vi "Initialize UI.vi"(8 "error in (no error)":errorcluster, 11 "UI in":refnum<class "UI.lvclass">) -> (0 "error out":errorcluster, 2 "stop event":refnum<user-event>, 3 "UI out":refnum<class "UI.lvclass">)   [LabVIEW 2016, in "Generic UI Actor.lvlib" / "UI.lvclass"]
uses:
  UI.lvclass
  UI.lvclass/UI.ctl
  Accessors/Write This VI.vi
  Accessors/Read This VI.vi
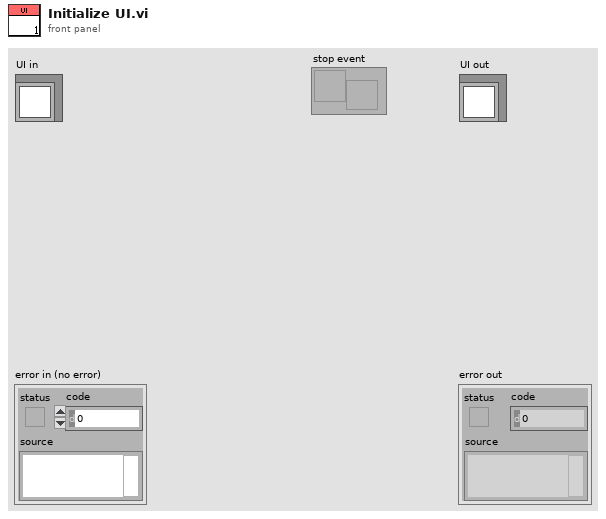
[diagram p1: front panel]
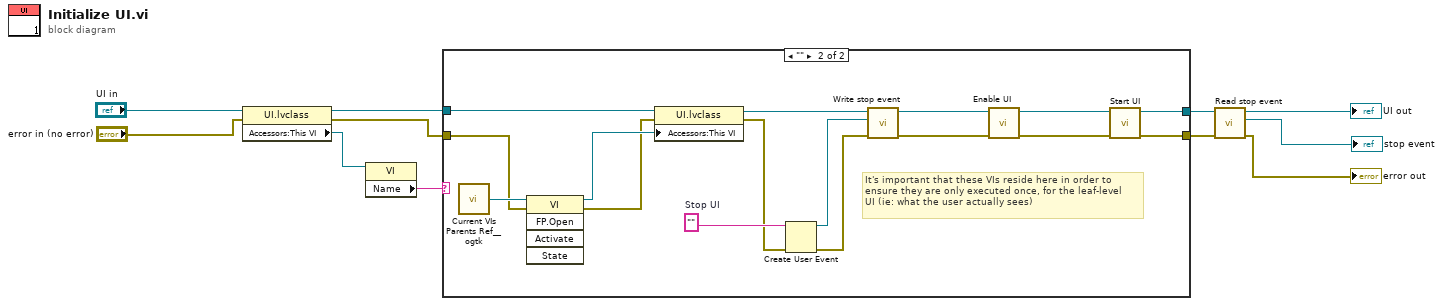
[diagram p0: block diagram]
diagram:
  n1 = property class="UI.lvclass"(reference="UI in", error in="error in (no error)") -> (reference out=w3:refnum<class "UI.lvclass">, error out=w1:errorcluster, "Accessors:This VI"=w2:refnum<vi>)
  n2 = property class="VI"(reference=w2) -> ("Name"=w11:string)  [unwired: 1 in, 2 out]
  n3 = case shown="\"\"" w11 {
    tunnel: [w12 w14] -> w10
    tunnel: w3 -> [w12 w24]
    tunnel: [w13 w15] -> w7
    tunnel: w1 -> [w13 w25]
    frame Default {
    }
    frame "" {
      w26 = ""  # Stop UI
      # "It's important that these VIs reside here in order to \nensure they are only executed once, for the leaf-level\nUI (ie: what the user actually sees)"
      n4 = call <userlib>:"Current VIs Parents Ref__ogtk.vi"() -> ("Calling VI's Reference"=w29:refnum<vi>)  [unwired: 2 in]
      n5 = invoke class="VI" method="FP.Open"(reference=w29, error in=w25) -> (reference out=w22:refnum<vi>, error out=w20:errorcluster)  [unwired: 3 in, 3 out]
      n6 = property class="UI.lvclass"(reference=w24, error in=w20, "Accessors:This VI"=w22) -> (reference out=w23:refnum<class "UI.lvclass">, error out=w21:errorcluster)
      n7 = Create User Event(user event datatype=w26, error in=w21) -> (user event=w27:refnum<user-event>, error out=w28:errorcluster)
      n8 = call "Write stop event.vi"("error in (no error)"=w28, "stop event"=w27, "UI in"=w23) -> ("error out"=w18:errorcluster, "UI out"=w19:refnum<class "UI.lvclass">)  [unwired: 7 in]
      n9 = call-dynamic "Enable UI.vi"("error in (no error)"=w18, "UI in"=w19) -> ("error out"=w16:errorcluster, "UI out"=w17:refnum<class "UI.lvclass">)  [unwired: 8 in]
      n10 = call-dynamic "Start UI.vi"("error in (no error)"=w16, "UI in"=w17) -> ("error out"=w15:errorcluster, "UI out"=w14:refnum<class "UI.lvclass">)  [unwired: 8 in]
    }
  }
  n11 = call "Read stop event.vi"("error in (no error)"=w7, "UI in"=w10) -> ("error out"=→"error out":errorcluster, "stop event"=→"stop event":refnum<user-event>, "UI out"=→"UI out":refnum<class "UI.lvclass">)  [unwired: 7 in]
